vi "determine winner.vi"(9 "Player2":dbl, 11 "Player1":dbl) -> (3 "Result":string)   [LabVIEW 2014]
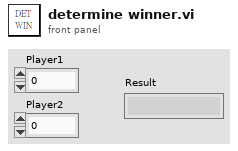
[diagram p1: front panel]
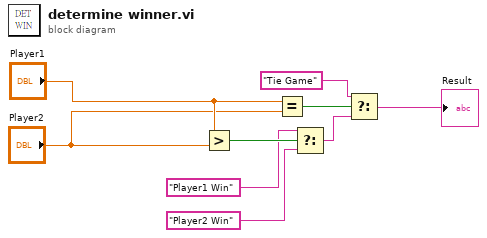
[diagram p0: block diagram]
diagram:
  n1 = Greater?(x="Player1", y="Player2") -> (0:w7:bool)
  n2 = Equal?(x="Player1", y="Player2") -> (x = y?=w9:bool)
  n3 = Select(t="Player1 Win" ("Player1Win"), s=w7, f="Player2 Win" ("Player2Win")) -> (s? t:f=w3:string)
  n4 = Select(t="Tie Game" ("Tie"), s=w9, f=w3) -> (s? t:f=→"Result":string)
